vi "String to Sorting Enum.vi"(8 "error in":errorcluster, 11 "string in":string) -> (0 "error out":errorcluster, 3 "Sorting":T1)   [LabVIEW 2018]
uses:
  Type Defs/Sorting Methods.ctl
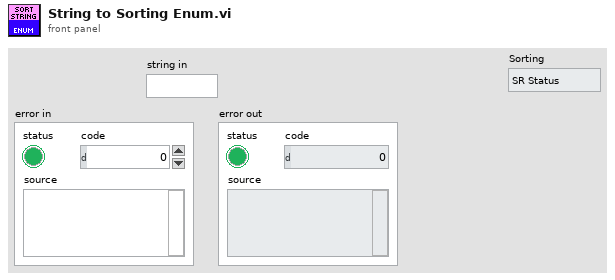
[diagram p1: front panel]
types:
  T1 = typedef "Sorting Methods.ctl" = enum16{"SR Status", "Most Recent", "SR Type", "SR Number"}
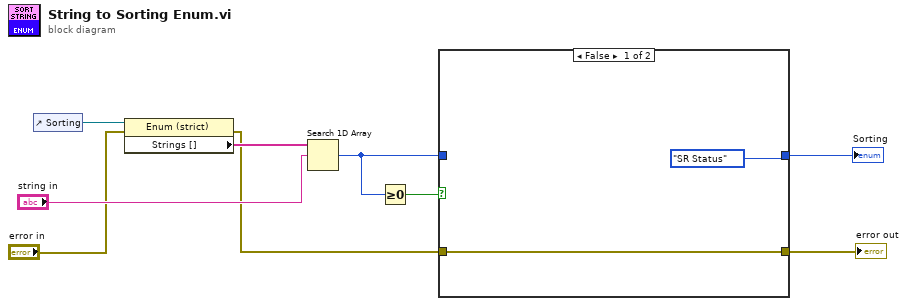
[diagram p0: block diagram]
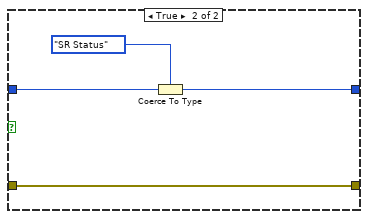
[diagram p2: hidden frame]
diagram:
  n1 = control-ref of="Sorting"() -> (w1:refnum<vi>)
  n2 = property class="Enum (strict)"(reference=w1, error in="error in") -> (error out=w4:errorcluster, "Strings []"=w9:string[])  [unwired: 1 out]
  n3 = Search 1D Array(1D array=w9, element="string in") -> (index of element=w7:i32)  [unwired: 1 in]
  n4 = Greater Or Equal To 0?(x=w7) -> (x >= 0?=w8:bool)
  n5 = case shown="False" w8 {
    tunnel: w7 -> [_ w15]
    tunnel: [Sorting_Methods."SR Status" ("Sorting") w14] -> w2
    tunnel: w4 -> [w11 w13]
    tunnel: [w11 w13] -> w3
    frame False {
    }
    frame True {
      n6 = Coerce To Type(0:w15, 1:Sorting_Methods."SR Status" ("Sorting")) -> (2:w14:T1)
    }
  }
  "error out" <- w3
  "Sorting" <- w2
